vi "Test - Selection List Target.vi"() -> ()   [LabVIEW 2023]
doc: "This VI is used by the Selected Objects and the Clipboard examples."
panel:
  in  "Cluster":cluster{"String":string}
  in  "Boolean":bool
  in  "Numeric":dbl
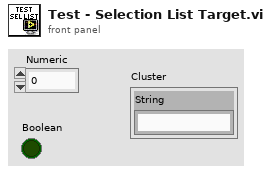
[diagram p1: front panel]
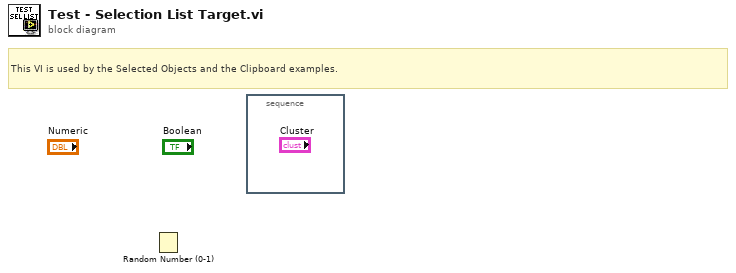
[diagram p0: block diagram]
diagram:
  # "This VI is used by the Selected Objects and the Clipboard examples."
  n1 = Random Number (0-1)() -> ()  [unwired: 1 out]
  n2 = stacked-sequence {
    frame #0 {
    }
  }
